vi "[GV]_Lidar Obstacle (거리제한).vi"() -> ()   [LabVIEW 2016, in "Lidar Variables.lvlib"]
uses:
  Lidar Variables.lvlib
panel:
  in  "Lidar Obstacle (거리제한)":dbl[][](array[numeric])
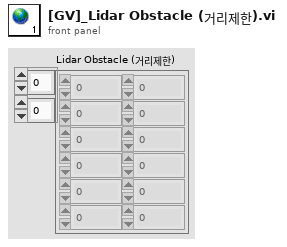
[diagram p1: front panel]
diagram:
